vi "StimLevel-Initialize.vi"(0 "Level":T1, 11 "error in (no error)":errorcluster) -> (4 "Level out":T1, 15 "error out":errorcluster)   [LabVIEW 2020]
uses:
  Controls/Level XCtl/Level Data.ctl
  Controls/Level XCtl/Level Units.ctl
  Controls/Level XCtl/Level XCtl.xctl
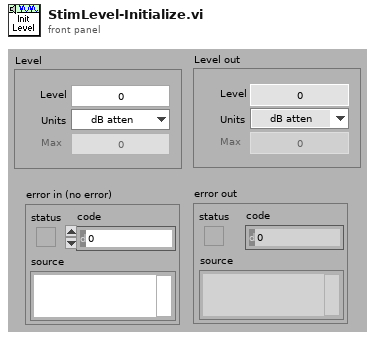
[diagram p1: front panel]
types:
  T1 = typedef "Level XCtl.xctl/Level Data.ctl" = cluster{"Level":dbl, "Units":T2, "Max":dbl, "Multiplier":dbl, "Cal File":path, "Cal":cluster{"Freq (Hz)":dbl[], "Mag (dB SPL)":dbl[], "Phase (deg)":dbl[]}}
  T2 = typedef "Level Units.ctl" = enum16{"dB atten", "dB SPL", "dB re 1 Vrms", "dB V/Hz½", "mW", "dB HL", "Volts", "dB mW"}
  T3 = cluster{"Frequency (Hz)":dbl[], "Mag":dbl[], "Phase":dbl[]}
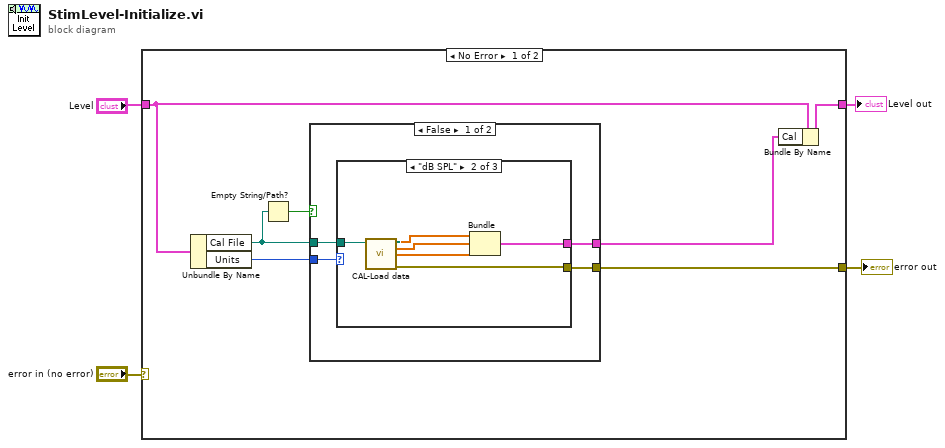
[diagram p0: block diagram]
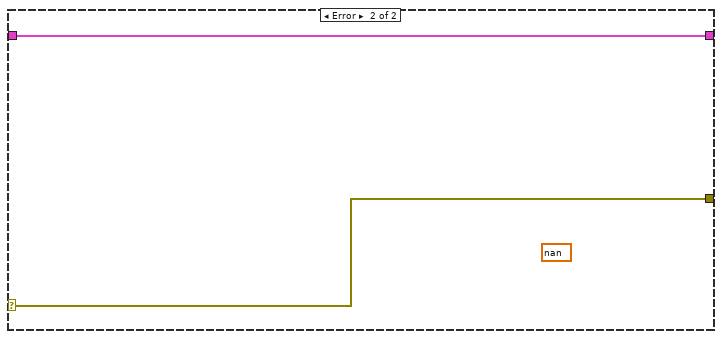
[diagram p5: hidden frame]
diagram:
  n1 = case shown="No Error" "error in (no error)" {
    selector: "error in (no error)" -> [_ w23]
    tunnel: "Level" -> [w10 w22]
    tunnel: [w11 w23] -> w3
    tunnel: [w9 w22] -> w1
    frame No Error {
      n2 = Unbundle By Name(w10) -> ("Cal File"=w5:path, "Units"=w8:T2)
      n3 = Empty String/Path?(string/path=w5) -> (empty?=w7:bool)
      n4 = case shown="False" w7 {
        tunnel: [w15 _] -> w11
        tunnel: w8 -> [w14 _]
        tunnel: w5 -> [w13 _]
        tunnel: [w12 _] -> w6
        frame False {
          n5 = case shown="\"dB SPL\"" w14 {
            tunnel: [_ w21 _] -> w15
            tunnel: w13 -> [_ w20 _]
            tunnel: [_ w16 _] -> w12
            frame "dB atten", Default {
            }
            frame "dB SPL" {
              n6 = call "CAL-Load data.vi"("user path"=w20) -> ("Frequency (Hz)"=w19:dbl[], "Mag"=w18:dbl[], "Phase"=w17:dbl[], "error out"=w21:errorcluster)  [unwired: 7 in, 4 out]
              n7 = Bundle("Frequency (Hz)"=w19, "Mag"=w18, "Phase"=w17) -> (w16:T3)  [unwired: 1 in]
            }
            frame "dB re 1 Vrms" {
            }
          }
        }
        frame True {
        }
      }
      n8 = Bundle By Name(cluster=w10, "Cal"=w6) -> (w9:T1)
    }
    frame Error {
      (unwired) nan ("Reference Level")
    }
  }
  "error out" <- w3
  "Level out" <- w1
